vi "Find and Call MeasurementLink Plugin.vi"() -> ()   [LabVIEW 2020]
uses:
  <vilib>/MeasurementLink/MeasurementLink Discovery Client/MeasurementLink Discovery Client.lvlib
  <vilib>/MeasurementLink/MeasurementLink Discovery Client/RPC Messages/ni_measurementlink_discovery_v1_EnumerateServicesRequest.ctl
  <vilib>/MeasurementLink/MeasurementLink Discovery Client/RPC Messages/ni_measurementlink_discovery_v1_ResolveServiceRequest.ctl
  <vilib>/gRPC/LabVIEW gRPC Library/grpc-lvsupport-release.lvlib
  045899de-a912-426a-8a5d-a949b9672173.vi
  Measurement Results.ctl
  MeasurementLink measurement_client/MeasurementLink measurement_client.lvlib
  MeasurementLink measurement_client/RPC Messages/google_protobuf_Any.ctl
  MeasurementLink measurement_client/RPC Messages/ni_measurementlink_PinMapContext.ctl
  MeasurementLink measurement_client/RPC Messages/ni_measurementlink_measurement_v1_MeasureRequest.ctl
  <vilib>/MeasurementLink/MeasurementLink Discovery Client/RPC Messages/ni_measurementlink_discovery_v1_ServiceLocation.ctl
  Measurement Configuration.ctl
panel:
  in  "stop":bool
  out "waveform graph":dbl[](graph)
  out "available services":string[](array[string])
  in  "measurement configuration":T1={"Frequency"=1.0, "Amplitude"=1.0}
  out "error out":errorcluster
  out "matched service":T2
  out "Found?":bool
  in  "address":string="localhost:42000"
  in  "service to run":string="GetSineSignal_LabVIEW"
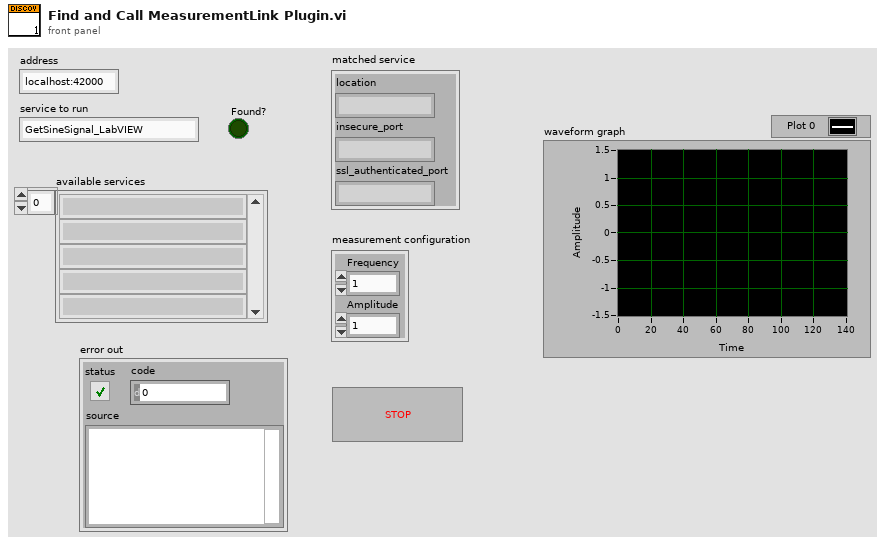
[diagram p1: front panel]
types:
  T1 = typedef "Measurement Configuration.ctl" = cluster{"Frequency":dbl, "Amplitude":dbl}
  T2 = typedef "MeasurementLink Discovery Client.lvlib/ni_measurementlink_discovery_v1_ServiceLocation.ctl" = cluster{"location":string, "insecure_port":string, "ssl_authenticated_port":string}
  T3 = typedef "Measurement Results.ctl" = cluster{"Array":dbl[]}
  T4 = typedef "MeasurementLink Discovery Client.lvlib/ni_measurementlink_discovery_v1_ResolveServiceRequest.ctl" = cluster{"provided_interface":string, "service_class":string}
  T5 = typedef "MeasurementLink Discovery Client.lvlib/ni_measurementlink_discovery_v1_EnumerateServicesRequest.ctl" = cluster{"provided_interface":string}
  T6 = typedef "grpc-lvsupport-release.lvlib/grpcId.ctl" = u64
  T7 = typedef "MeasurementLink Discovery Client.lvlib/ni_measurementlink_discovery_v1_EnumerateServicesResponse.ctl" = cluster{"available_services":T8[]}
  T8 = typedef "MeasurementLink Discovery Client.lvlib/ni_measurementlink_discovery_v1_ServiceDescriptor.ctl" = cluster{"display_name":string, "description_url":string, "provided_interfaces":string[], "service_class":string, "annotations":T9[]}
  T9 = typedef "MeasurementLink Discovery Client.lvlib/ni_measurementlink_discovery_v1_ServiceDescriptor_AnnotationsEntry.ctl" = cluster{"key":string, "value":string}
  T10 = typedef "grpc-lvsupport-release.lvlib/Message Metadata.ctl" = cluster{"Version":i32, "Name":string, "Type Url":string, "Elements":T11[], "Has Oneof":bool}
  T11 = typedef "grpc-lvsupport-release.lvlib/Message Element Metadata.ctl" = cluster{"Field Name":string, "Embedded Message Name":string, "Protobuf Index":i32, "MessageElementType":T12, "Repeated":bool, "Is in Oneof":bool, "Oneof Container Name":string}
  T12 = typedef "grpc-lvsupport-release.lvlib/Message Element Type.ctl" = enum32{"Int32Value", "FloatValue", "DoubleValue", "BoolValue", "StringValue", "MessageValue", "Int64Value", "UInt32Value", "UInt64Value", "EnumValue", "Bytes", "Fixed64", "Fixed32", "SFixed64", "SFixed32", "SInt64", "SInt32"}
  T13 = typedef "MeasurementLink measurement_client.lvlib/ni_measurementlink_measurement_v1_MeasureRequest.ctl" = cluster{"configuration_parameters":T14, "pin_map_context":T15}
  T14 = typedef "MeasurementLink measurement_client.lvlib/google_protobuf_Any.ctl" = cluster{"type_url":string, "value":u8[]}
  T15 = typedef "MeasurementLink measurement_client.lvlib/ni_measurementlink_PinMapContext.ctl" = cluster{"pin_map_id":string, "sites":i32[]}
  T16 = typedef "grpc-lvsupport-release.lvlib/Any.ctl" = cluster{"Type Url":string, "Bytes":u8[]}
  T17 = typedef "MeasurementLink measurement_client.lvlib/ni_measurementlink_measurement_v1_MeasureResponse.ctl" = cluster{"outputs":T14}
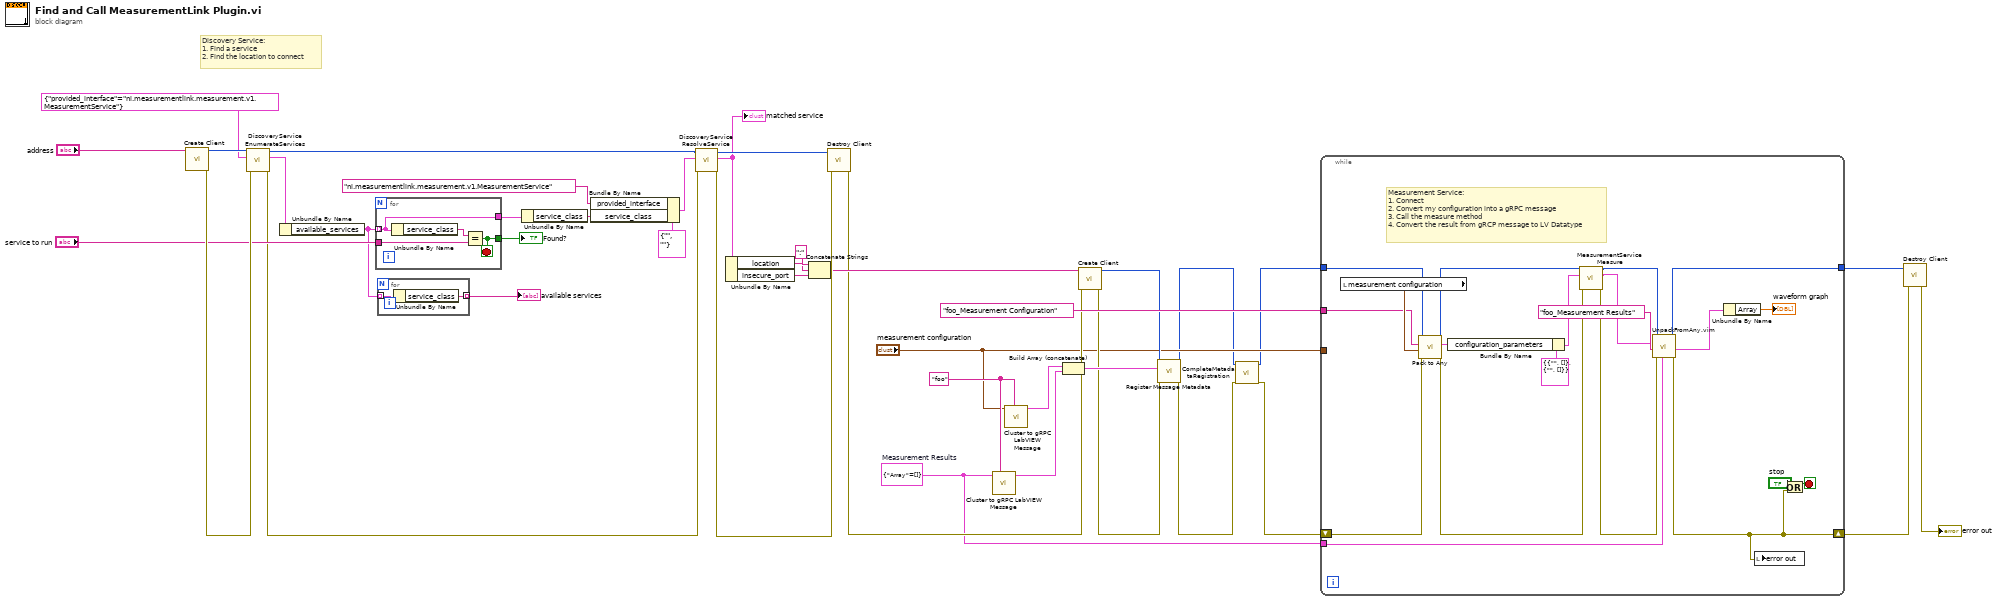
[diagram p0: block diagram]
diagram:
  w6 = T3 {"Array"=[]}  # Measurement Results
  w18 = "foo" ("Package Name")
  # "Discovery Service:\n1. Find a service\n2. Find the location to connect"
  n1 = call <vilib>:"Create Client.vi"("address"="address") -> ("error out"=w38:errorcluster, "gRPC ID Out"=w39:T6)  [unwired: 9 in]
  n2 = call <vilib>:"DiscoveryService EnumerateServices.vi"("error in"=w38, "Request Data"=T5 {"provided_interface"="ni.measurementlink.measurement.v1.MeasurementService"}, "gRPC ID"=w39) -> ("error out"=w31:errorcluster, "Response Data"=w36:T7, "gRPC ID out"=w32:T6)  [unwired: 6 in]
  n3 = Unbundle By Name(w36) -> ("available_services"=w17:T8[])
  n4 = for {
    tunnel: w17 -> [w42] mode=indexing
    tunnel: "service to run" -> [w43]
    tunnel: [w42] -> w33
    tunnel: [w41] -> w34
    stop <- w41 stop-if-true
    n5 = Unbundle By Name(w42) -> ("service_class"=w44:string)
    n6 = Equal?(x=w44, y=w43) -> (x = y?=w41:bool)
  }
  "Found?" <- w34
  n7 = for {
    tunnel: w17 -> [w46] mode=indexing
    tunnel: [w45] -> w16 mode=indexing
    n8 = Unbundle By Name(w46) -> ("service_class"=w45:string)
  }
  "available services" <- w16
  n9 = Unbundle By Name(w33) -> ("service_class"=w27:string)
  n10 = Bundle By Name(cluster=T4 {"provided_interface"="", "service_class"=""} ("Request Data"), "provided_interface"="ni.measurementlink.measurement.v1.MeasurementService", "service_class"=w27) -> (w25:T4)
  n11 = call <vilib>:"DiscoveryService ResolveService.vi"("error in"=w31, "Request Data"=w25, "gRPC ID"=w32) -> ("error out"=w30:errorcluster, "Response Data"=w24:T2, "gRPC ID out"=w29:T6)  [unwired: 6 in]
  "matched service" <- w24
  n12 = Unbundle By Name(w24) -> ("location"=w23:string, "insecure_port"=w21:string)
  n13 = Concatenate Strings(w23, ":" ("string"), w21) -> (w13:string)
  n14 = call <vilib>:"Destroy Client.vi"("error in"=w30, "gRPC ID"=w29) -> ("error out"=w12:errorcluster)  [unwired: 9 in]
  n15 = call <vilib>:"Cluster to gRPC LabVIEW Message.vi"("Package Name"=w18, "Cluster"=w6) -> ("gRPC Message Metadata []"=w19:T10[])  [unwired: 7 in, 2 out]
  n16 = call <vilib>:"Cluster to gRPC LabVIEW Message.vi"("Package Name"=w18, "Cluster"="measurement configuration") -> ("gRPC Message Metadata []"=w20:T10[])  [unwired: 7 in, 2 out]
  n17 = Build Array (concatenate)(w20, w19) -> (w15:T10[])
  n18 = call <vilib>:"Create Client.vi"("error in"=w12, "address"=w13) -> ("error out"=w11:errorcluster, "gRPC ID Out"=w10:T6)  [unwired: 8 in]
  n19 = call <vilib>:"Register Message Metadata.vi"("error in"=w11, "Messages"=w15, "gRPCid in"=w10) -> ("error out"=w2:errorcluster, "gRPCid out"=w4:T6)  [unwired: 7 in]
  n20 = call <vilib>:"CompleteMetadataRegistration.vi"("error in"=w2, "gRPC ID in"=w4) -> ("error out"=w1:errorcluster, "gRPC ID Out"=w3:T6)  [unwired: 8 in]
  n21 = while {
    tunnel: w3 -> [w50]
    tunnel: "foo_Measurement Configuration" ("Message Type") -> [w47]
    tunnel: [w64] -> w9
    tunnel: "measurement configuration" -> [_]
    shift-right: [w52] -> w8
    shift-left: w1 -> [w65]
    tunnel: w6 -> [w55]
    stop <- w53 stop-if-true
    # "Measurement Service:\n1. Connect\n2. Convert my configuration into a gRPC message\n3. Call the measure method\n4. Convert the result from gRCP message to LV Datatype"
    n22 = local read "measurement configuration"() -> (w51:T1)
    n23 = call "Pack to Any.vi"("error in"=w65, "Data To Pack"=w51, "Message Type"=w47, "gRPCid in"=w50) -> ("error out"=w49:errorcluster, "Any"=w48:T16, "gRPCid out"=w63:u64)  [unwired: 5 in]
    n24 = Bundle By Name(cluster=T13 {"configuration_parameters"={"type_url"="", "value"=[]}, "pin_map_context"={"pin_map_id"="", "sites"=[]}} ("Request Data"), "configuration_parameters"=w48) -> (w59:T13)
    n25 = call "MeasurementService Measure.vi"("error in"=w49, "Request Data"=w59, "gRPC ID"=w63) -> ("error out"=w61:errorcluster, "Response Data"=w54:T17, "gRPC ID out"=w62:T6)  [unwired: 6 in]
    n26 = call "UnpackFromAny.vim"("Data Type"=w55, "error in"=w61, "Message Type"="foo_Measurement Results", "Any"=w54, "gRPCid in"=w62) -> ("error out"=w52:errorcluster, "Unpacked Value"=w56:T3, "gRPCid out"=w64:u64)  [unwired: 4 in]
    n27 = Unbundle By Name(w56) -> ("Array"=→"waveform graph":dbl[])
    n28 = local write "error out"(w52) -> ()
    n29 = Or(x="stop", y=w52) -> (x .or. y?=w53:bool)
  }
  n30 = call <vilib>:"Destroy Client.vi"("error in"=w8, "gRPC ID"=w9) -> ("error out"=→"error out":errorcluster)  [unwired: 9 in]
